vi "Cal_Calculations.vi"(1 "Error In":errorcluster) -> (0 "Error Out":errorcluster)   [LabVIEW 2019]
uses:
  Global Variables/Global_Variables.vi
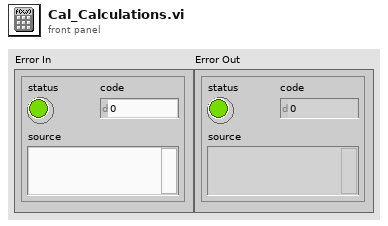
[diagram p1: front panel]
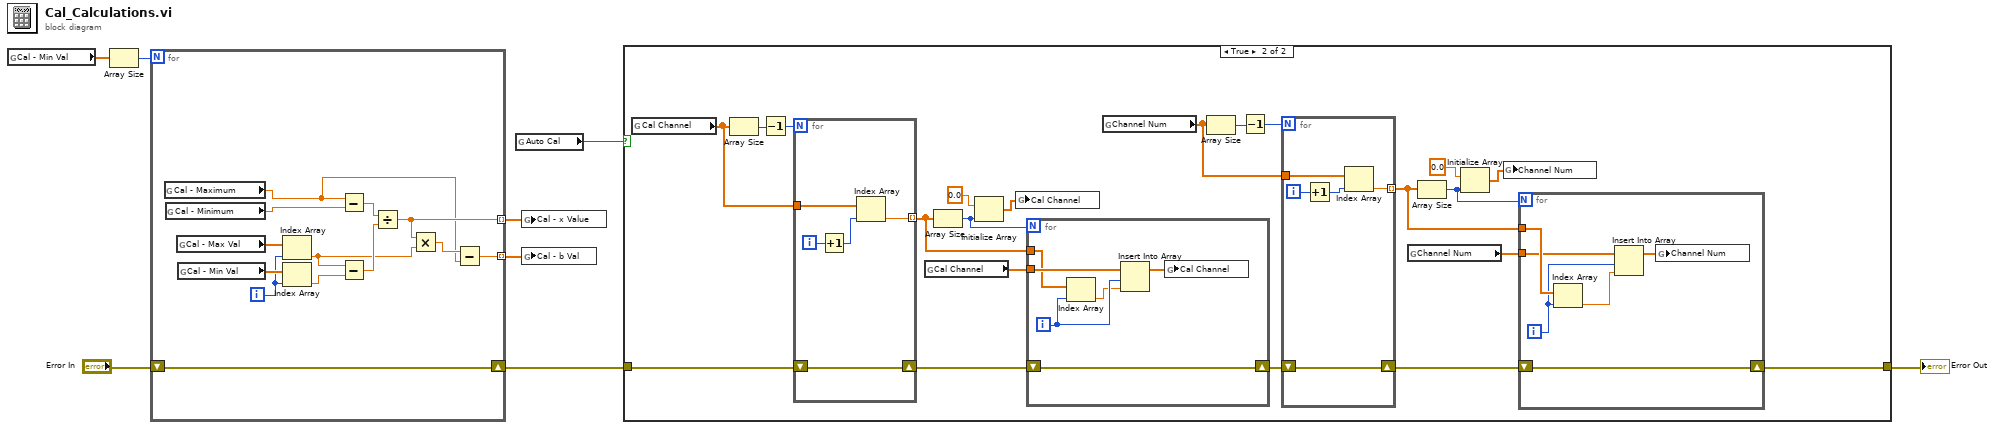
[diagram p0: block diagram]
diagram:
  n1 = global read "Global_Variables.vi" "Cal - Min Val"() -> (w6:dbl[])
  n2 = Array Size(array=w6) -> (size(s)=w7:i32)
  n3 = for {
    N: w7 -> [_]
    shift-right: [w9] -> w2
    shift-left: "Error In" -> [w9]
    tunnel: [w13] -> w4 mode=indexing
    tunnel: [w10] -> w5 mode=indexing
    i -> [w19]
    n4 = global read "Global_Variables.vi" "Cal - Maximum"() -> (w11:dbl)
    n5 = global read "Global_Variables.vi" "Cal - Minimum"() -> (w18:dbl)
    n6 = global read "Global_Variables.vi" "Cal - Max Val"() -> (w21:dbl[])
    n7 = global read "Global_Variables.vi" "Cal - Min Val"() -> (w20:dbl[])
    n8 = Index Array(array=w21, index=w19) -> (element=w14:dbl)
    n9 = Index Array(array=w20, index=w19) -> (element=w17:dbl)
    n10 = Subtract(x=w11, y=w18) -> (x-y=w16:dbl)
    n11 = Subtract(x=w14, y=w17) -> (x-y=w15:dbl)
    n12 = Divide(x=w16, y=w15) -> (x/y=w13:dbl)
    n13 = Multiply(x=w13, y=w14) -> (x*y=w12:dbl)
    n14 = Subtract(x=w12, y=w11) -> (x-y=w10:dbl)
  }
  n15 = global read "Global_Variables.vi" "Auto Cal"() -> (w3:bool)
  n16 = global write "Global_Variables.vi" "Cal - x Value"(w4) -> ()
  n17 = global write "Global_Variables.vi" "Cal - b Val"(w5) -> ()
  n18 = case shown="True" w3 {
    tunnel: w2 -> [w22 w43]
    tunnel: [w22 w23] -> w1
    frame False {
    }
    frame True {
      n19 = global read "Global_Variables.vi" "Cal Channel"() -> (w40:dbl[])
      n20 = Array Size(array=w40) -> (size(s)=w42:i32)
      n21 = Decrement(x=w42) -> (x-1=w41:i32)
      n22 = for {
        N: w41 -> [_]
        shift-right: [w64] -> w35
        shift-left: w43 -> [w64]
        tunnel: w40 -> [w62]
        tunnel: [w61] -> w30 mode=indexing
        i -> [w65]
        n23 = Increment(x=w65) -> (x+1=w63:i32)
        n24 = Index Array(array=w62, index=w63) -> (element=w61:dbl)
      }
      n25 = global read "Global_Variables.vi" "Cal Channel"() -> (w31:dbl[])
      n26 = Array Size(array=w30) -> (size(s)=w34:i32)
      n27 = Initialize Array(0.0 ("element"), w34) -> (w32:dbl[])
      n28 = global write "Global_Variables.vi" "Cal Channel"(w32) -> ()
      n29 = for {
        N: w34 -> [_]
        shift-right: [w55] -> w33
        shift-left: w35 -> [w55]
        tunnel: w31 -> [w53]
        tunnel: w30 -> [w52]
        i -> [w51]
        n30 = Index Array(array=w52, index=w51) -> (element=w50:dbl)
        n31 = Insert Into Array(array=w53, index=w51, new element=w50) -> (w54:dbl[])
        n32 = global write "Global_Variables.vi" "Cal Channel"(w54) -> ()
      }
      n33 = global read "Global_Variables.vi" "Channel Num"() -> (w37:dbl[])
      n34 = Array Size(array=w37) -> (size(s)=w39:i32)
      n35 = Decrement(x=w39) -> (x-1=w38:i32)
      n36 = for {
        N: w38 -> [_]
        shift-right: [w57] -> w24
        shift-left: w33 -> [w57]
        tunnel: w37 -> [w59]
        tunnel: [w56] -> w27 mode=indexing
        i -> [w60]
        n37 = Increment(x=w60) -> (x+1=w58:i32)
        n38 = Index Array(array=w59, index=w58) -> (element=w56:dbl)
      }
      n39 = global read "Global_Variables.vi" "Channel Num"() -> (w26:dbl[])
      n40 = Array Size(array=w27) -> (size(s)=w28:i32)
      n41 = Initialize Array(0.0, w28) -> (w25:dbl[])
      n42 = global write "Global_Variables.vi" "Channel Num"(w25) -> ()
      n43 = for {
        N: w28 -> [_]
        tunnel: w27 -> [w49]
        tunnel: w26 -> [w48]
        shift-right: [w45] -> w23
        shift-left: w24 -> [w45]
        i -> [w46]
        n44 = Index Array(array=w49, index=w46) -> (element=w47:dbl)
        n45 = Insert Into Array(array=w48, index=w46, new element=w47) -> (w44:dbl[])
        n46 = global write "Global_Variables.vi" "Channel Num"(w44) -> ()
      }
    }
  }
  "Error Out" <- w1
